vi "Actor Core.vi"(8 "error in":errorcluster caption="错误输入", 11 "VoiceControl in":refnum<class "Voice.lvclass"> caption="操作者输入") -> (0 "error out":errorcluster caption="错误输出", 3 "Actor out":refnum<class "Actor.lvclass"> caption="操作者输出")   [LabVIEW 2014, in "Voice.lvlib" / "Voice.lvclass"]
doc: "(<B>文件名</B>：Actor Framework.lvlib:Actor.lvclass:Actor Core.vi)\n\n接收发送至操作者的消息，响应消息并处理可能导致操作者关闭的错误。\n\n子孙类重写该VI，使操作者完成特定的任务。使用调用父方法节点实现重写。"
uses:
  Voice.lvclass
  <vilib>/ActorFramework/Actor/Actor.lvclass
  <vilib>/ActorFramework/Actor/Actor.lvclass/Actor.ctl
  Voice.lvclass/Voice.ctl
  <vilib>/Utility/tcp.llb/UDP Multicast Read-Only Open.vi
  <vilib>/regexp/Match Regular Expression.xnode
panel:
  out "standard error":string caption="命令行执行错误"
  out "error out 2":errorcluster caption="Python执行错误"
  out "格式化机器人指令":string[][](array[string])
  out "语音信号输出字符串":string
  in  "停止信号":bool
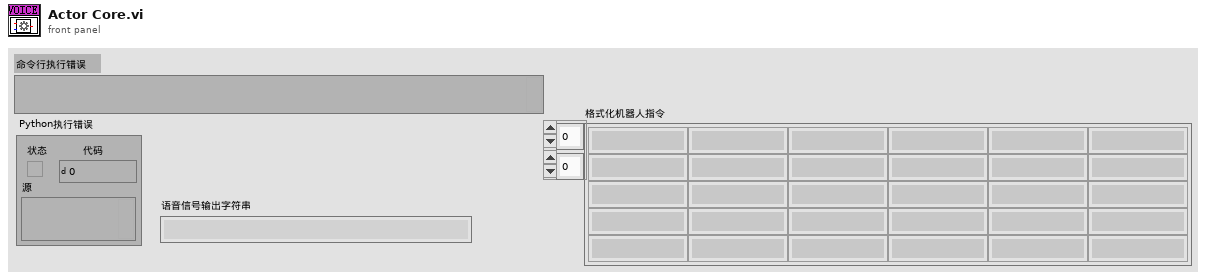
[diagram p1: front panel]
types:
  T1 = cluster{"Stop":refnum<user-event>, "Text":refnum<user-event>, "Connected":refnum<user-event>}
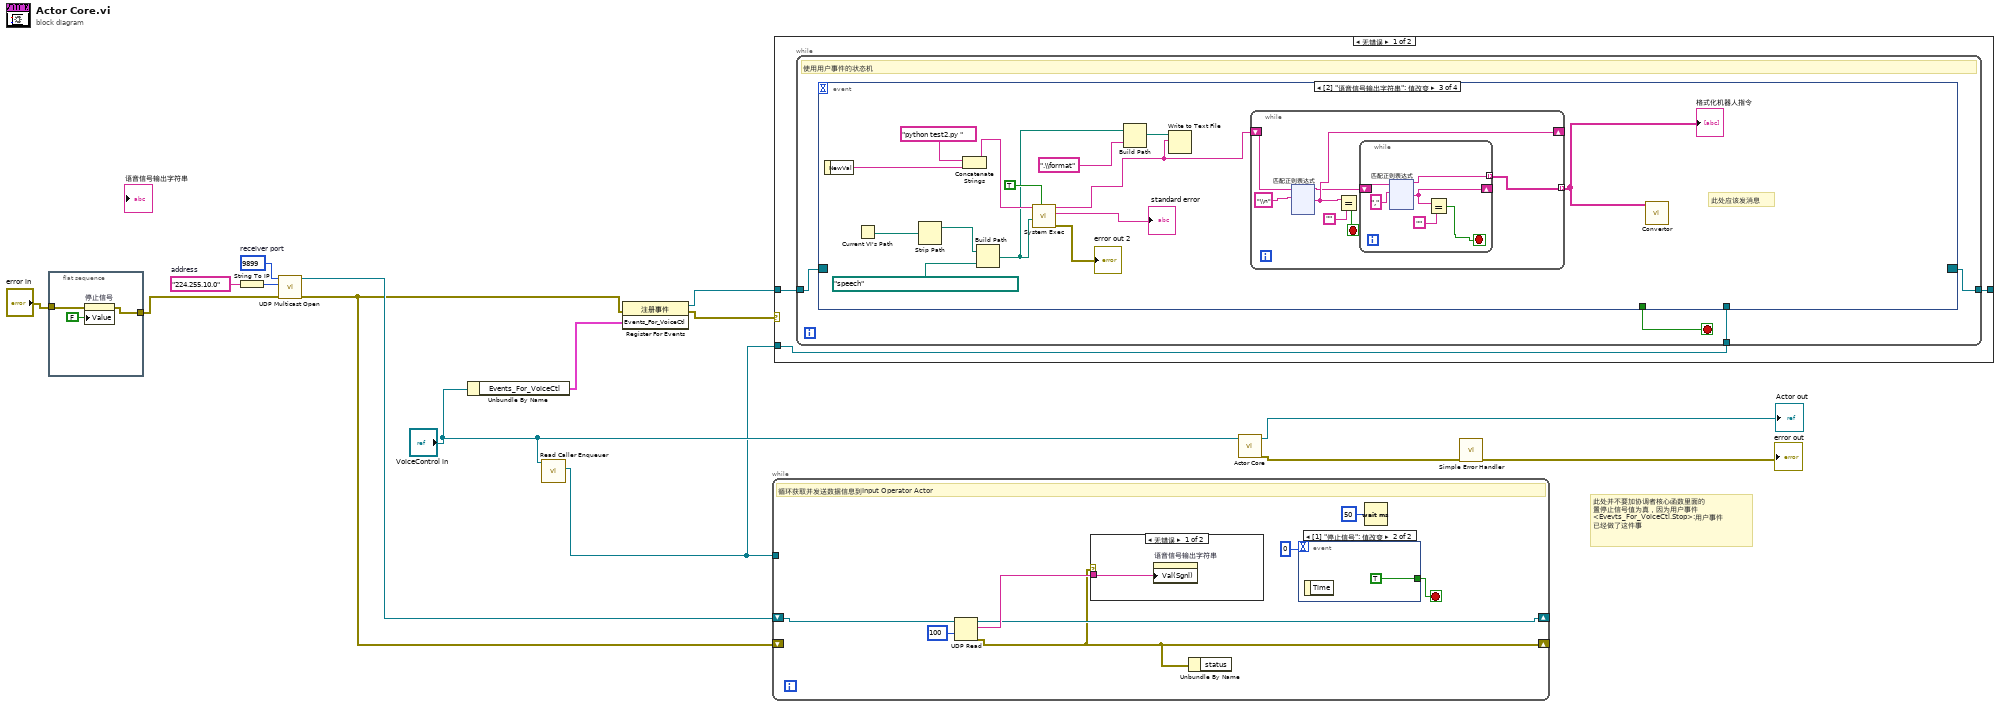
[diagram p0: block diagram]
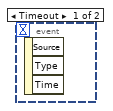
[diagram p3: hidden frame]
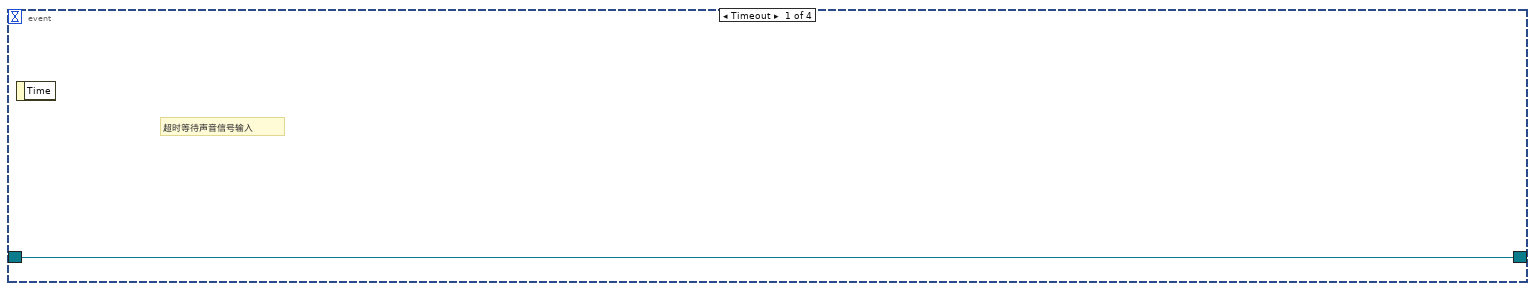
[diagram p4: hidden frame]
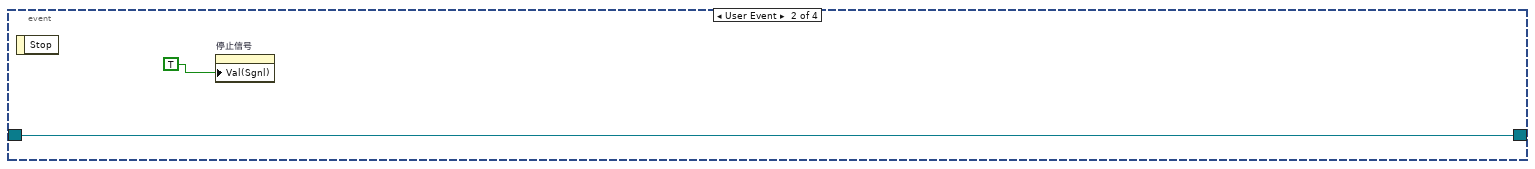
[diagram p5: hidden frame]
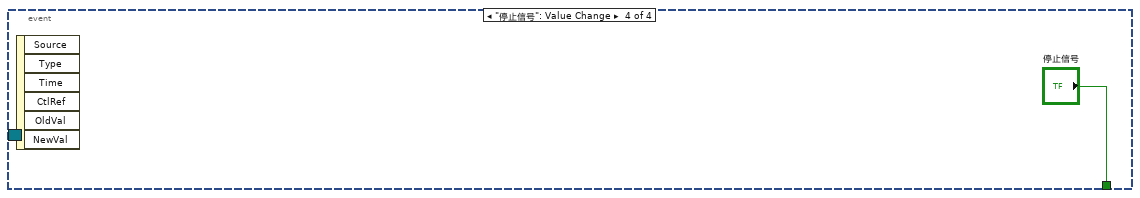
[diagram p6: hidden frame]
diagram:
  w7 = u16 9899  # receiver port
  w6 = "224.255.10.0"  # address
  # "此处并不要加协调者核心函数里面的\n置停止信号值为真，因为用户事件\n<Evevts_For_VoiceCtl.Stop>:用户事件\n已经做了这件事"
  n1 = flat-sequence {
    tunnel: "error in" -> [w18]
    tunnel: [w16] -> w5
    frame #0 {
      n2 = property on="停止信号" class="Bool (严格)"(error in=w18, "Value"=FALSE ("停止信号")) -> (error out=w16:errorcluster)  [unwired: 1 in, 1 out]
    }
  }
  n3 = String To IP(1:w6) -> (0:w8:u32)
  n4 = call-poly <vilib>:"UDP Multicast Open.vi"("error in (no error)"=w5, "multicast addr"=w8, "port"=w7) -> ("error out"=w3:errorcluster, "connection ID"=w4:refnum<k16>)  [unwired: 6 in, 1 out]
  n5 = Unbundle By Name("VoiceControl in") -> ("Events_For_VoiceCtl"=w14:T1)
  n6 = call <vilib>:"Read Caller Enqueuer.vi"("Actor"="VoiceControl in") -> ("Caller Enqueuer"=w1:refnum<class "Message Enqueuer.lvclass">)  [unwired: 10 in]
  n7 = register-events(error in=w3, w14) -> (reference out=w13:refnum<event-registration>, error out=w11:errorcluster)  [unwired: 1 in]
  n8 = while {
    tunnel: w1 -> [_]
    shift-right: [w20] -> _
    shift-left: w4 -> [w21]
    shift-right: [w19] -> _
    shift-left: w3 -> [_]
    stop <- w24 stop-if-true
    # "循环获取并发送数据信息到Input Operator Actor"
    n9 = UDP Read(connection ID=w21, timeout ms (25000)=100 ("超时毫秒(25000)")) -> (data out=w23:string, error out=w19:errorcluster, 3:w20:refnum<k16>)  [unwired: 1 in, 3 out]
    n10 = case shown="无错误" w19 {
      tunnel: w23 -> [w27 _]
      frame No Error {
        n11 = property on="语音信号输出字符串" class="Str"("Val(Sgnl)"=w27) -> ()  [unwired: 2 in, 2 out]
      }
      frame Error {
      }
    }
    n12 = Unbundle By Name(w19) -> ()  [unwired: 1 out]
    n13 = event shown="[1] \"停止信号\": 值改变" {
      selector: _ -> [_ _]
      dyn-events: _ -> [_ _]
      timeout: 0 -> [_ _]
      tunnel: [_ TRUE] -> w24
      event Timeout {
        n14 = event-data() -> ()  [unwired: 1 in, 3 out]
      }
      event "停止信号": Value Change {
        n15 = event-data() -> ()  [unwired: 1 in, 1 out]
      }
    }
    n16 = Wait (ms)(milliseconds to wait=u32 50 ("等待时间（毫秒）")) -> ()  [unwired: 1 out]
  }
  n17 = case shown="无错误" w11 {
    tunnel: [w31 w295] -> _
    tunnel: w13 -> [w30 w295]
    tunnel: w1 -> [w29 _]
    frame No Error {
      n18 = while {
        tunnel: [w34] -> w31
        tunnel: w30 -> [w33]
        tunnel: w29 -> [w32]
        stop <- w35 stop-if-true
        # "使用用户事件的状态机"
        n19 = event shown="[2] \"语音信号输出字符串\": 值改变" {
          selector: w33 -> [w36 w38 _ _]
          dyn-events: [w36 w38 _ _] -> w34
          timeout: _ -> [_ _ _ _]
          tunnel: [_ _ _ "停止信号"] -> w35
          tunnel: w32 -> [_ _ _ _]
          event Timeout {
            # "超时等待声音信号输入"
            n20 = event-data() -> ()  [unwired: 1 in, 1 out]
          }
          event User Event {
            n21 = event-data() -> ()  [unwired: 1 in, 1 out]
            n22 = property on="停止信号" class="Bool (严格)"("Val(Sgnl)"=TRUE) -> ()  [unwired: 2 in, 2 out]
          }
          event "语音信号输出字符串": Value Change {
            # "此处应该发消息"
            n23 = event-data() -> ("NewVal"=w44:string)  [unwired: 1 in]
            n24 = Current VI's Path() -> (path=w39:path)
            n25 = Strip Path(path=w39) -> (stripped path=w42:path)  [unwired: 1 out]
            n26 = Concatenate Strings("python test2.py " ("command line"), w44) -> (w49:string)
            n27 = Build Path(base path=w42, name or relative path=path "speech") -> (appended path=w41:path)
            n28 = call <vilib>:"System Exec.vi"("wait until completion? (T)"=TRUE, "working directory"=w41, "command line"=w49) -> ("error out"=→"error out 2":errorcluster, "standard error"=→"standard error":string, "standard output"=w52:string)  [unwired: 5 in, 1 out]
            n29 = Build Path(base path=w41, name or relative path=".\\format" ("名称或相对路径")) -> (appended path=w51:path)
            n30 = Write to Text File(file (use dialog)=w51, text=w52) -> ()  [unwired: 2 in, 3 out]
            n31 = while {
              tunnel: [w53] -> w40 mode=indexing
              shift-right: [w57] -> _
              shift-left: w52 -> [w58]
              stop <- w55 stop-if-true
              n32 = xnode "匹配正则表达式"("输入字符串"=w58, "正则表达式"="\\n") -> ("匹配之前"=w54:string, "匹配之后"=w57:string)  [unwired: 4 in, 3 out]
              n33 = Equal?(x=w57, y="") -> (x = y?=w55:bool)
              n34 = while {
                shift-right: [w61] -> _
                shift-left: w54 -> [w65]
                tunnel: [w63] -> w53 mode=indexing
                stop <- w60 stop-if-true
                n35 = xnode "匹配正则表达式"("输入字符串"=w65, "正则表达式"=",") -> ("匹配之前"=w63:string, "匹配之后"=w61:string)  [unwired: 4 in, 3 out]
                n36 = Equal?(x=w61, y="") -> (x = y?=w60:bool)
              }
            }
            "格式化机器人指令" <- w40
            n37 = call "Convertor.vi"("机器人指令数组"=w40) -> ()  [unwired: 10 in, 1 out]
          }
          event "停止信号": Value Change {
            n38 = event-data() -> ()  [unwired: 1 in, 6 out]
          }
        }
      }
    }
    frame Error {
    }
  }
  n39 = call-parent "Actor Core.vi"("Actor in"="VoiceControl in") -> ("error out"=w9:errorcluster, "Actor out"=→"Actor out":refnum<class "Actor.lvclass">)  [unwired: 9 in]
  n40 = call <vilib>:"Simple Error Handler.vi"("error in (no error)"=w9) -> ("error out"=→"error out":errorcluster)  [unwired: 4 in, 4 out]
